vi "VoltToCelcius.vi"(10 "Voltage":dbl) -> (2 "Temperature[C]":dbl)   [LabVIEW 2019]
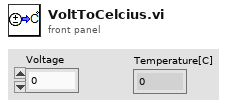
[diagram p1: front panel]
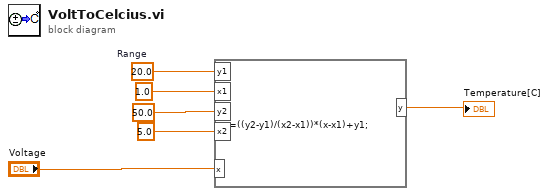
[diagram p0: block diagram]
diagram:
  w6 = 20.0  # Range
  n1 = formula code="y=((y2-y1)/(x2-x1))*(x-x1)+y1;"("x"="Voltage", "y1"=w6, "x1"=1.0 ("input variable"), "y2"=50.0 ("input variable"), "x2"=5.0 ("input variable")) -> ("y"=→"Temperature[C]":dbl)
